vi "Initialise devices.vi"() -> (5 "Number of connected devices":u32, 6 "Device handles":u64[](array[numeric]), 7 "Laser comms. error":errorcluster[](array[cluster]), 8 "Get lasers serial num. error":errorcluster, 9 "Device detection error":errorcluster, 10 "Device initialisation errors":errorcluster[](array[cluster]))   [LabVIEW 2018]
uses:
  Commands.ctl
  Coherent global.vi
panel:
  # "PN 05/11/2014\n      08/04/2019"
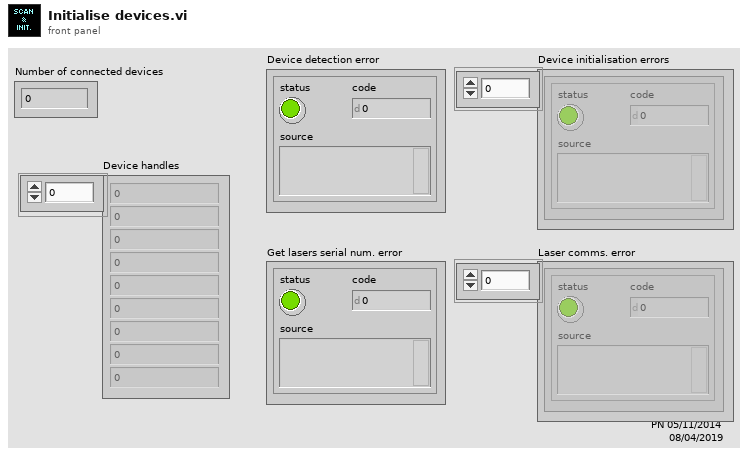
[diagram p1: front panel]
types:
  T1 = typedef "Commands.ctl" = u8
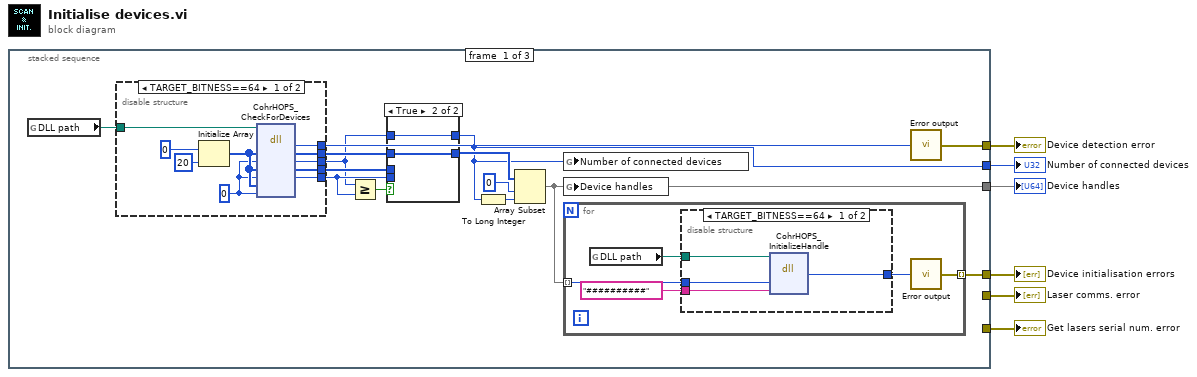
[diagram p0: block diagram]
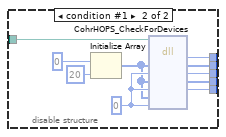
[diagram p2: hidden frame]
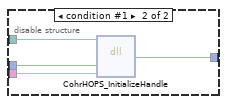
[diagram p4: hidden frame]
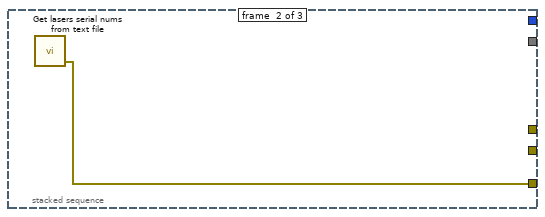
[diagram p5: hidden frame]
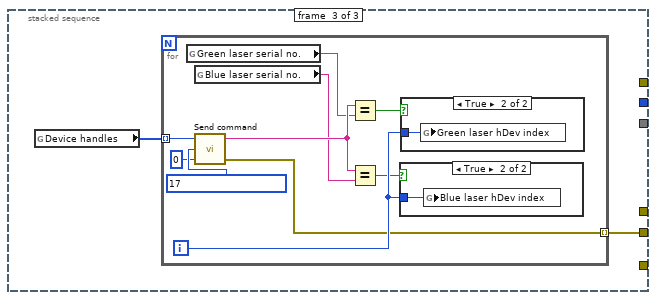
[diagram p6: hidden frame]
diagram:
  n1 = stacked-sequence {
    tunnel: [w17 _ _] -> w6
    tunnel: [w16 _ _] -> w5
    tunnel: [w15 _ _] -> w4
    tunnel: [w7 _ _] -> w3
    tunnel: [_ w58 _] -> w2
    tunnel: [_ _ w59] -> w1
    frame #0 {
      n2 = global read "Coherent global.vi" "DLL path"() -> (w14:path)
      n3 = disable-structure shown="TARGET_BITNESS==64" {
        disable-tunnel: [w25 w40] -> w18
        disable-tunnel: w14 -> [w26 w35]
        disable-tunnel: [w24 w34] -> w12
        disable-tunnel: [w22 w33] -> w11
        disable-tunnel: [w21 w32] -> w10
        disable-tunnel: [w23 w31] -> w9
        frame condition #0 (active) {
          w27 = u32 0 ("Input Value")
          n4 = Initialize Array(u64 0 ("Input Value"), 20 ("dimension size")) -> (w30:u64[])
          n5 = dll-call lib="?" fn="CohrHOPS_CheckForDevices"(path in=w26, "devicesConnected"=w30, "numberOfDevicesConnected"=w27, "devicesAdded"=w30, "numberOfDevicesAdded"=w27, "devicesRemoved"=w30, "numberOfDevicesRemoved"=w27) -> ("return value"=w25:i32, "devicesConnected"=w24:u64[], "numberOfDevicesConnected"=w23:u32, "devicesAdded"=w22:u64[], "numberOfDevicesAdded"=w21:u32)  [unwired: 4 in, 2 out]
        }
        frame condition #1 {
          w39 = u32 0 ("Input Value")
          n6 = Initialize Array(u32 0 ("Input Value"), 20 ("dimension size")) -> (w36:u32[])
          n7 = dll-call lib="?" fn="CohrHOPS_CheckForDevices"(path in=w35, "devicesConnected"=w36, "numberOfDevicesConnected"=w39, "devicesAdded"=w36, "numberOfDevicesAdded"=w39, "devicesRemoved"=w36, "numberOfDevicesRemoved"=w39) -> ("return value"=w40:i32, "devicesConnected"=w34:u32[], "numberOfDevicesConnected"=w31:u32, "devicesAdded"=w33:u32[], "numberOfDevicesAdded"=w32:u32)  [unwired: 4 in, 2 out]
        }
      }
      n8 = Greater Or Equal?(x=w9, y=w10) -> (x >= y?=w13:bool)
      n9 = case shown="True" w13 {
        tunnel: w12 -> [_ w43]
        tunnel: w11 -> [w42 _]
        tunnel: w10 -> [w41 _]
        tunnel: w9 -> [_ w44]
        tunnel: [w41 w44] -> w7
        tunnel: [w42 w43] -> w8
        frame False {
        }
        frame True {
        }
      }
      n10 = To Long Integer(number=w7) -> (32bit integer=w20:i32)
      n11 = Array Subset(array=w8, index=0, length=w20) -> (w17:u64[])
      n12 = global write "Coherent global.vi" "Number of connected devices"(w7) -> ()
      n13 = global write "Coherent global.vi" "Device handles"(w17) -> ()
      n14 = for {
        tunnel: w17 -> [w49] mode=indexing
        tunnel: [w47] -> w15 mode=indexing
        n15 = global read "Coherent global.vi" "DLL path"() -> (w45:path)
        n16 = disable-structure shown="TARGET_BITNESS==64" {
          disable-tunnel: w49 -> [w50 w56]
          disable-tunnel: [w53 w54] -> w48
          disable-tunnel: "##########" ("headType") -> [w52 w55]
          disable-tunnel: w45 -> [w51 w57]
          frame condition #0 (active) {
            n17 = dll-call lib="?" fn="CohrHOPS_InitializeHandle"(path in=w51, "handle"=w50, "headType"=w52) -> ("return value"=w53:i32)  [unwired: 4 in, 2 out]
          }
          frame condition #1 {
            n18 = dll-call lib="?" fn="CohrHOPS_InitializeHandle"(path in=w57, "handle"=w56, "headType"=w55) -> ("return value"=w54:i32)  [unwired: 4 in, 2 out]
          }
        }
        n19 = call "Error output.vi"("I32 err code"=w48) -> ("Error Out"=w47:errorcluster)
      }
      n20 = call "Error output.vi"("I32 err code"=w18) -> ("Error Out"=w16:errorcluster)
    }
    frame #1 {
      n21 = call "Get lasers serial nums from text file.vi"() -> ("Error"=w58:errorcluster)  [unwired: 2 in, 2 out]
    }
    frame #2 {
      n22 = global read "Coherent global.vi" "Device handles"() -> (w60:u64[])
      n23 = for {
        tunnel: w60 -> [w69] mode=indexing
        tunnel: [w67] -> w59 mode=indexing
        i -> [w70]
        n24 = global read "Coherent global.vi" "Green laser serial no."() -> (w64:string)
        n25 = global read "Coherent global.vi" "Blue laser serial no."() -> (w65:string)
        n26 = call "Send command.vi"("Value"=u16 0, "Command"=T1 17, "Device handle"=w69) -> ("Error"=w67:errorcluster, "response"=w66:string)  [unwired: 1 out]
        n27 = Equal?(x=w66, y=w64) -> (x = y?=w63:bool)
        n28 = Equal?(x=w66, y=w65) -> (x = y?=w62:bool)
        n29 = case shown="True" w62 {
          tunnel: w70 -> [_ w72]
          frame False {
          }
          frame True {
            n30 = global write "Coherent global.vi" "Blue laser hDev index"(w72) -> ()
          }
        }
        n31 = case shown="True" w63 {
          tunnel: w70 -> [_ w71]
          frame False {
          }
          frame True {
            n32 = global write "Coherent global.vi" "Green laser hDev index"(w71) -> ()
          }
        }
      }
    }
  }
  "Device handles" <- w6
  "Device detection error" <- w5
  "Device initialisation errors" <- w4
  "Number of connected devices" <- w3
  "Get lasers serial num. error" <- w2
  "Laser comms. error" <- w1
